vi "Send Read Header.vi"(8 "error in (no error)":errorcluster, 11 "TCP Receive in":refnum<class "TCP Receive.lvclass">) -> (0 "error out":errorcluster, 3 "TCP Receive out":refnum<class "TCP Receive.lvclass">)   [LabVIEW 2020, in "TCP Receive.lvclass"]
uses:
  TCP Receive.lvclass
  <vilib>/addons/_Workers/Library/Classes/Message/Message.lvclass
  <vilib>/addons/_Workers/Library/Classes/Message/Enqueue Message to Self.vi
  C:/Program Files (x86)/National Instruments/LabVIEW 2020/vi.lib/addons/_Workers/Library/Classes/Worker User/Worker User.lvclass
  C:/Program Files (x86)/National Instruments/LabVIEW 2020/vi.lib/addons/_Workers/Library/Classes/Worker/Worker.lvclass
  C:/Program Files (x86)/National Instruments/LabVIEW 2020/vi.lib/addons/_Workers/Library/Classes/Workers Object/Workers Object.lvclass
  C:/Users/TestAdmin/git/TCP-Workers/Workers/TCP Receive/TCP Receive.lvclass
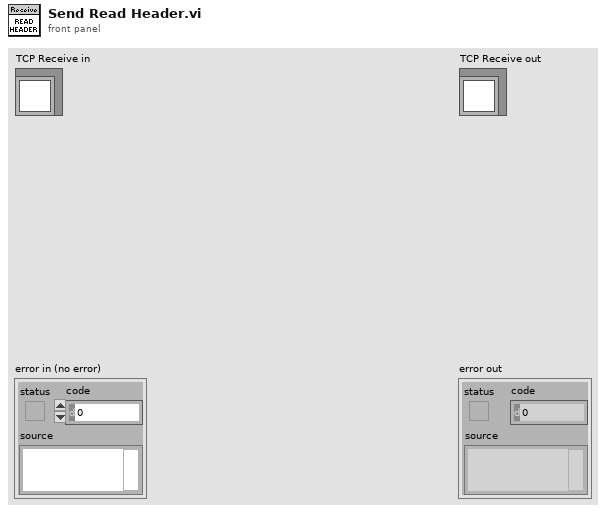
[diagram p1: front panel]
types:
  T1 = typedef "Workers.lvlib/Case Label.ctl" = string
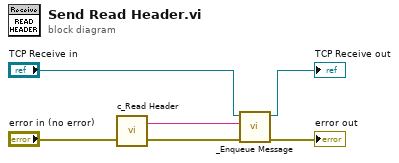
[diagram p0: block diagram]
diagram:
  n1 = call "c_Read Header.vi"() -> ("Case Label"=w5:T1)  [unwired: 1 in]
  n2 = call-poly <vilib>:"_Enqueue Message.vi"("error in"="error in (no error)", "Case Label"=w5, "Worker"="TCP Receive in") -> ("error out"=→"error out":errorcluster, "dup Worker out"=→"TCP Receive out":refnum<class "TCP Receive.lvclass">)  [unwired: 7 in]
